vi "MakeTiff.vi"(2 "z":i32, 3 "X":i32, 4 "Y":i32, 5 "file path":path) -> (0 "error out":errorcluster, 1 "refnum tif":refnum<file>)   [LabVIEW 2014]
panel:
  out "size(s)":i32
  out "appended array":u16[](array[numeric])
  out "x*y":i32
  out "IFDend":u32
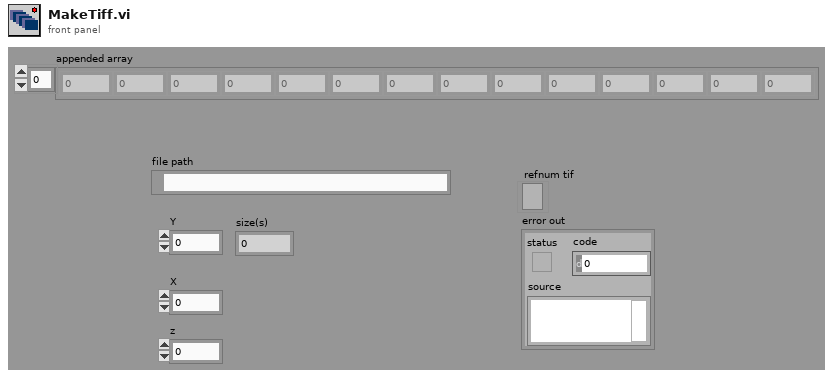
[diagram p1: front panel]
types:
  T1 = enum16{"open", "replace", "create", "open or create", "replace or create", "replace or create with confirmation"}
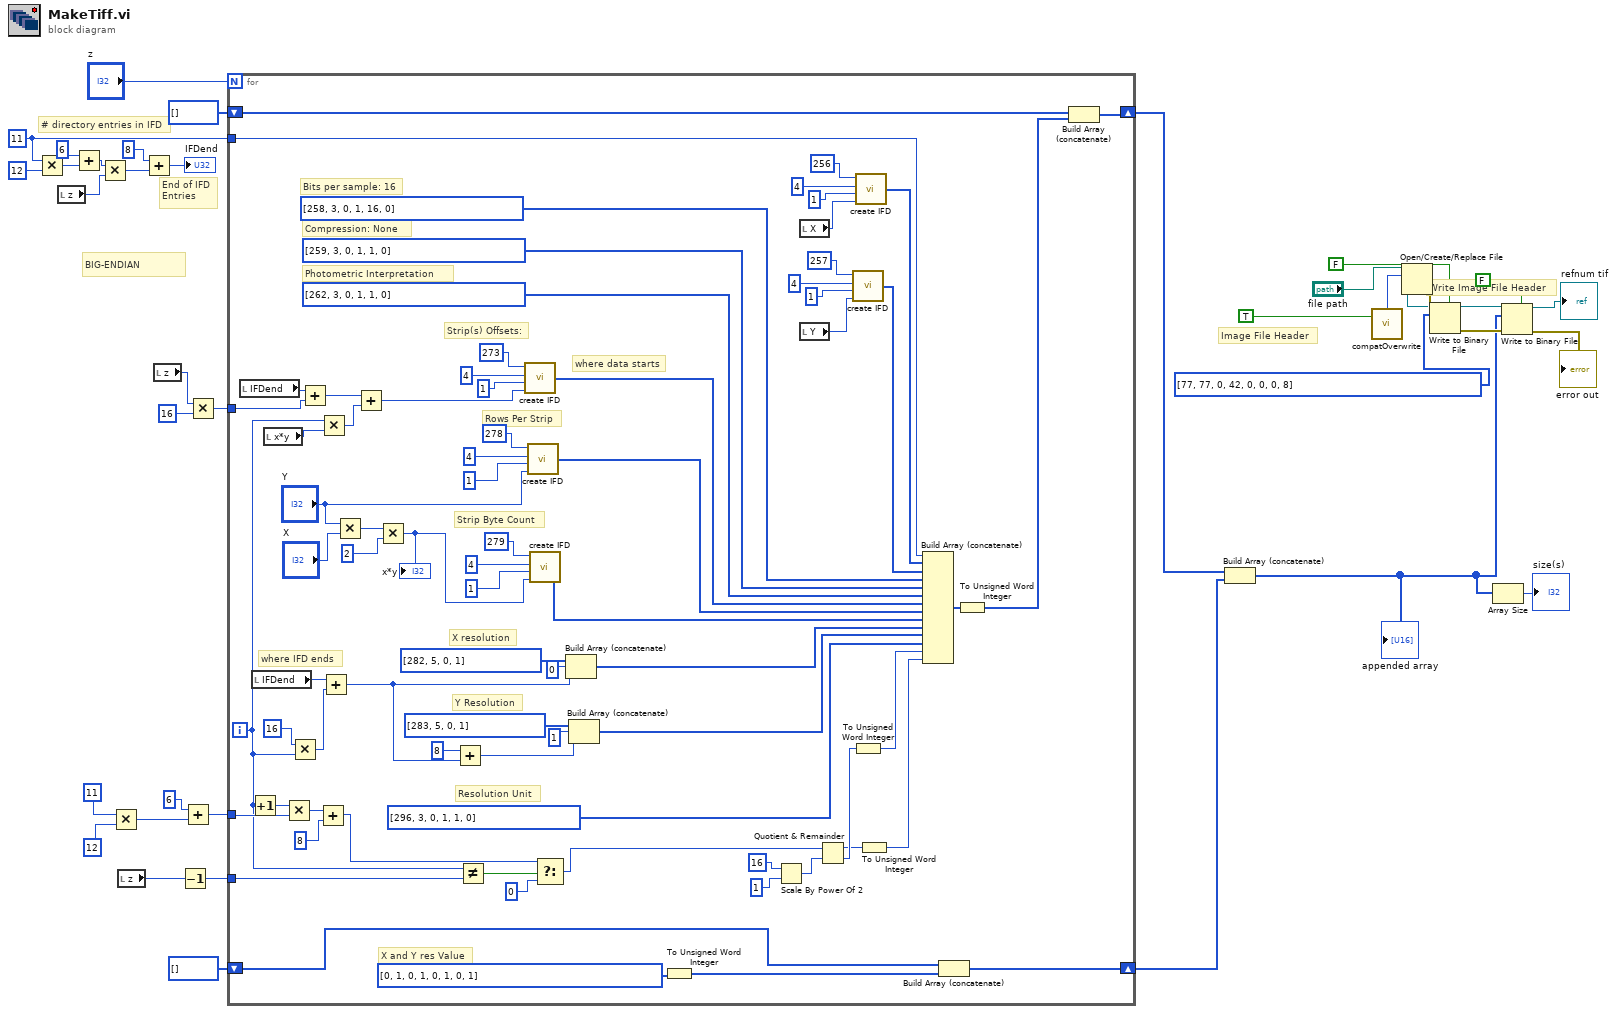
[diagram p0: block diagram]
diagram:
  w30 = u16 11
  # "Image File Header"
  # "Write Image File Header"
  # "End of IFD\nEntries"
  # "# directory entries in IFD"
  # "BIG-ENDIAN"
  n1 = Multiply(x=w30, y=u16 12) -> (x*y=w29:u16)
  n2 = local read "z"() -> (w20:i32)
  n3 = Add(x=u16 6, y=w29) -> (x+y=w23:u16)
  n4 = Multiply(x=w23, y=w20) -> (x*y=w35:i32)
  n5 = Multiply(x=11, y=12) -> (x*y=w25:i32)
  n6 = local read "z"() -> (w18:i32)
  n7 = Add(x=8, y=w35) -> (x+y=→"IFDend":i32)
  n8 = local read "z"() -> (w19:i32)
  n9 = Decrement(x=w18) -> (x-1=w21:i32)
  n10 = Add(x=u16 6, y=w25) -> (x+y=w24:i32)
  n11 = Multiply(x=w19, y=16) -> (x*y=w31:i32)
  n12 = for {
    N: "z" -> [_]
    shift-right: [w67] -> w16
    shift-left: u16[] [] -> [w80]
    shift-right: [w77] -> w15
    shift-left: u16[] [] -> [w76]
    tunnel: w30 -> [w75]
    tunnel: w31 -> [w70]
    tunnel: w24 -> [w64]
    tunnel: w21 -> [w60]
    i -> [w59]
    # "where IFD ends"
    # "where data starts"
    # "X and Y res Value"
    # "Resolution Unit"
    # "Y Resolution"
    # "X resolution"
    # "Bits per sample: 16"
    # "Strip Byte Count"
    # "Rows Per Strip"
    # "Strip(s) Offsets:"
    # "Photometric Interpretation"
    # "Compression: None"
    n13 = local read "IFDend"() -> (w95:u32)
    n14 = Increment(x=w59) -> (x+1=w56:i32)
    n15 = local read "IFDend"() -> (w74:u32)
    n16 = local read "x*y"() -> (w53:i32)
    n17 = Multiply(x=w56, y=w64) -> (x*y=w63:i32)
    n18 = Multiply(x=16, y=w59) -> (x*y=w72:i32)
    n19 = Add(x=w95, y=w70) -> (x+y=w69:u32)
    n20 = Add(x=w63, y=8) -> (x+y=w61:i32)
    n21 = Multiply(x=w59, y=w53) -> (x*y=w68:i32)
    n22 = Add(x=w74, y=w72) -> (x+y=w73:u32)
    n23 = Multiply(x="Y", y="X") -> (x*y=w50:i32)
    n24 = Add(x=w69, y=w68) -> (x+y=w66:u32)
    n25 = Multiply(x=w50, y=2) -> (x*y=w49:i32)
    "x*y" <- w49
    n26 = Add(x=u32 8, y=w73) -> (x+y=w65:u32)
    n27 = Not Equal?(x=w59, y=w60) -> (x != y?=w58:bool)
    n28 = call "create IFD.vi"("Value/Offset"=w66, "Count"=u32 1, "TYPE"=u16 4, "TAG"=u16 273) -> ("IFD entry"=w89:u16[])
    n29 = call "create IFD.vi"("Value/Offset"="Y", "Count"=u32 1, "TYPE"=u16 4, "TAG"=u16 278) -> ("IFD entry"=w88:u16[])
    n30 = call "create IFD.vi"("Value/Offset"=w49, "Count"=u32 1, "TYPE"=u16 4, "TAG"=u16 279) -> ("IFD entry"=w87:u16[])
    n31 = Select(t=w61, s=w58, f=u16 0) -> (s? t:f=w42:i32)
    n32 = Build Array (concatenate)(u16[] [282, 5, 0, 1], 0, w73) -> (w86:u32[])
    n33 = Build Array (concatenate)(u16[] [283, 5, 0, 1], 1, w65) -> (w85:u32[])
    n34 = To Unsigned Word Integer(number=u16[] [0, 1, 0, 1, 0, 1, 0, 1]) -> (unsigned 16bit integer=w78:u16[])
    n35 = Scale By Power Of 2(n=u32 16, x=u32 1) -> (x*2^n=w45:u32)
    n36 = local read "X"() -> (w54:i32)
    n37 = local read "Y"() -> (w55:i32)
    n38 = Quotient & Remainder(x=w42, y=w45) -> (x-y*floor(x/y)=w43:u32, floor(x/y)=w44:u32)
    n39 = call "create IFD.vi"("Value/Offset"=w55, "Count"=u32 1, "TYPE"=u16 4, "TAG"=u16 257) -> ("IFD entry"=w93:u16[])
    n40 = To Unsigned Word Integer(number=w44) -> (unsigned 16bit integer=w40:u16)
    n41 = call "create IFD.vi"("Value/Offset"=w54, "Count"=u32 1, "TYPE"=u16 4, "TAG"=u16 256) -> ("IFD entry"=w94:u16[])
    n42 = To Unsigned Word Integer(number=w43) -> (unsigned 16bit integer=w39:u16)
    n43 = Build Array (concatenate)(w75, w94, w93, u16[] [258, 3, 0, 1, 16, 0], u16[] [259, 3, 0, 1, 1, 0], u16[] [262, 3, 0, 1, 1, 0], w89, w88, w87, w86, w85, u16[] [296, 3, 0, 1, 1, 0], w40, w39) -> (w83:u32[])
    n44 = Build Array (concatenate)(w76, w78) -> (w77:u16[])
    n45 = To Unsigned Word Integer(number=w83) -> (unsigned 16bit integer=w41:u16[])
    n46 = Build Array (concatenate)(w80, w41) -> (w67:u16[])
  }
  n47 = Build Array (concatenate)(w16, w15) -> (w2:u16[])
  "appended array" <- w2
  n48 = call <vilib>:"compatOverwrite.vi"("overwrite (F)"=TRUE) -> ("overwrite?"=w3:T1)
  n49 = Open/Create/Replace File(file path (use dialog)="file path", operation (0:open)=w3) -> (refnum out=w8:refnum<file>, error out=w11:errorcluster)  [unwired: 1 in, 4 out]
  n50 = Write to Binary File(file (use dialog)=w8, data=u8[] [77, 77, 0, 42, 0, 0, 0, 8], error in=w11, 5:FALSE ("prepend array or string size? (T)")) -> (refnum out=w9:refnum<file>, error out=w10:errorcluster)  [unwired: 3 out]
  n51 = Array Size(array=w2) -> (size(s)=→"size(s)":i32)
  n52 = Write to Binary File(file (use dialog)=w9, data=w2, error in=w10, 5:FALSE ("prepend array or string size? (T)")) -> (refnum out=→"refnum tif":refnum<file>, error out=→"error out":errorcluster)  [unwired: 3 out]
